vi "Nufern Functional Global.vi"(4 "Galvo.lvclass":refnum<class "Galvo.lvclass">, 7 "Nufern Functional\n Global States":T2, 8 "Error In":errorcluster, 10 "Nufern Digital Timing Control":T1={"Fire"=FALSE, "Start A-Scan"=0, "Stop A-Scan"=0, "Reps per Fire"=1, "B-Scan Spacing"=1} {"B-Scan Spacing" min=0 max=5000; "Reps per Fire" min=1 max=5000}) -> (0 "Error Out":errorcluster)   [LabVIEW 2015]
uses:
  Nufern Functional Global States.ctl
  Galvo/Galvo.lvclass
  Nufern Digital Timing Control.ctl
  NuFern.lvclass
  DIO/NIDIO/NIDIO.lvclass
panel:
  out "Waveform Graph":dbl[][](graph)
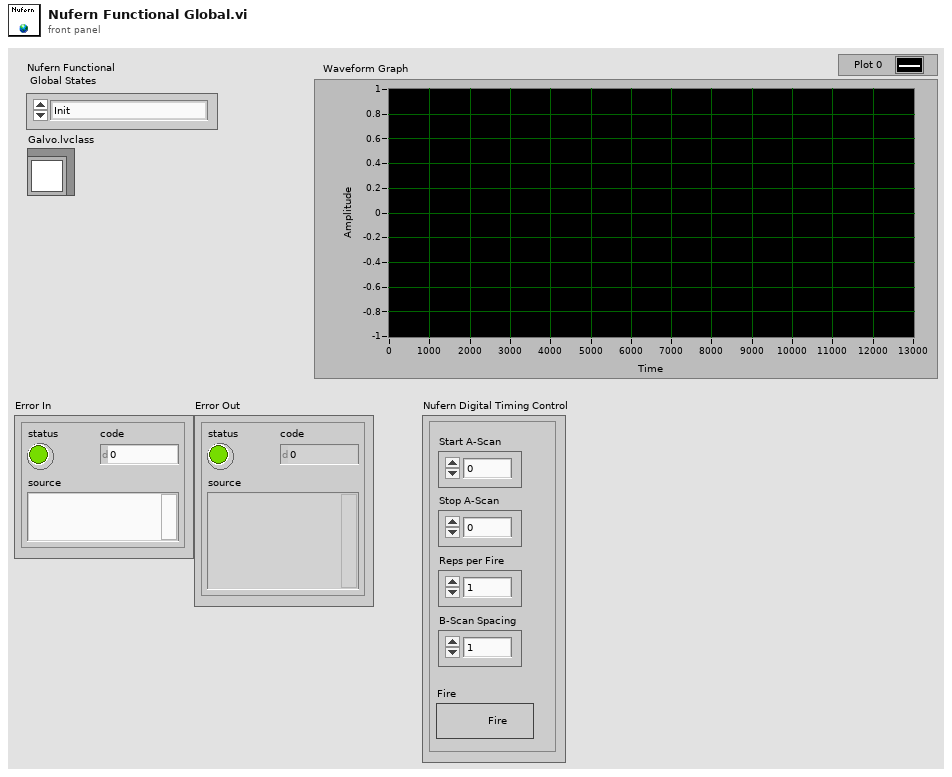
[diagram p1: front panel]
types:
  T1 = typedef "Nufern Digital Timing Control.ctl" = cluster{"Fire":bool, "Start A-Scan":u32, "Stop A-Scan":u32, "Reps per Fire":i32, "B-Scan Spacing":i32}
  T2 = typedef "Nufern Functional Global States.ctl" = enum16{"Init", "Generate Waveform", "Fire", "Shutdown", "Stop"}
  T3 = typedef "DAQ Class.lvclass/DAQ Parameters.ctl" = cluster{"Points Per A-Scan":u32, "A-Scans Per B-Scan":u32, "Number of B-Scans":u32, "B-Scans Per Transfer":u32, "Trigger Voltage":sgl, "Trigger Source":T4, "Trigger Slope":T5, "Channel":T6, "Clock":T7, "Bits per Sample":dbl, "Range":dbl, "Start Trim":u32, "Stop Trim":u32}
  T4 = typedef "DAQ Class.lvclass/Trigger Source.ctl" = enum16{"External", "Channel A", "Channel B"}
  T5 = typedef "DAQ Class.lvclass/Trigger Slope.ctl" = enum16{"Rising", "Falling"}
  T6 = typedef "OCT DAQ Channel Data Type.ctl" = enum16{"Channel 1", "Channel 2", "Channel 1 and 2"}
  T7 = typedef "DAQ Class.lvclass/Clock Control.ctl" = enum16{"Internal Clock", "External Clock"}
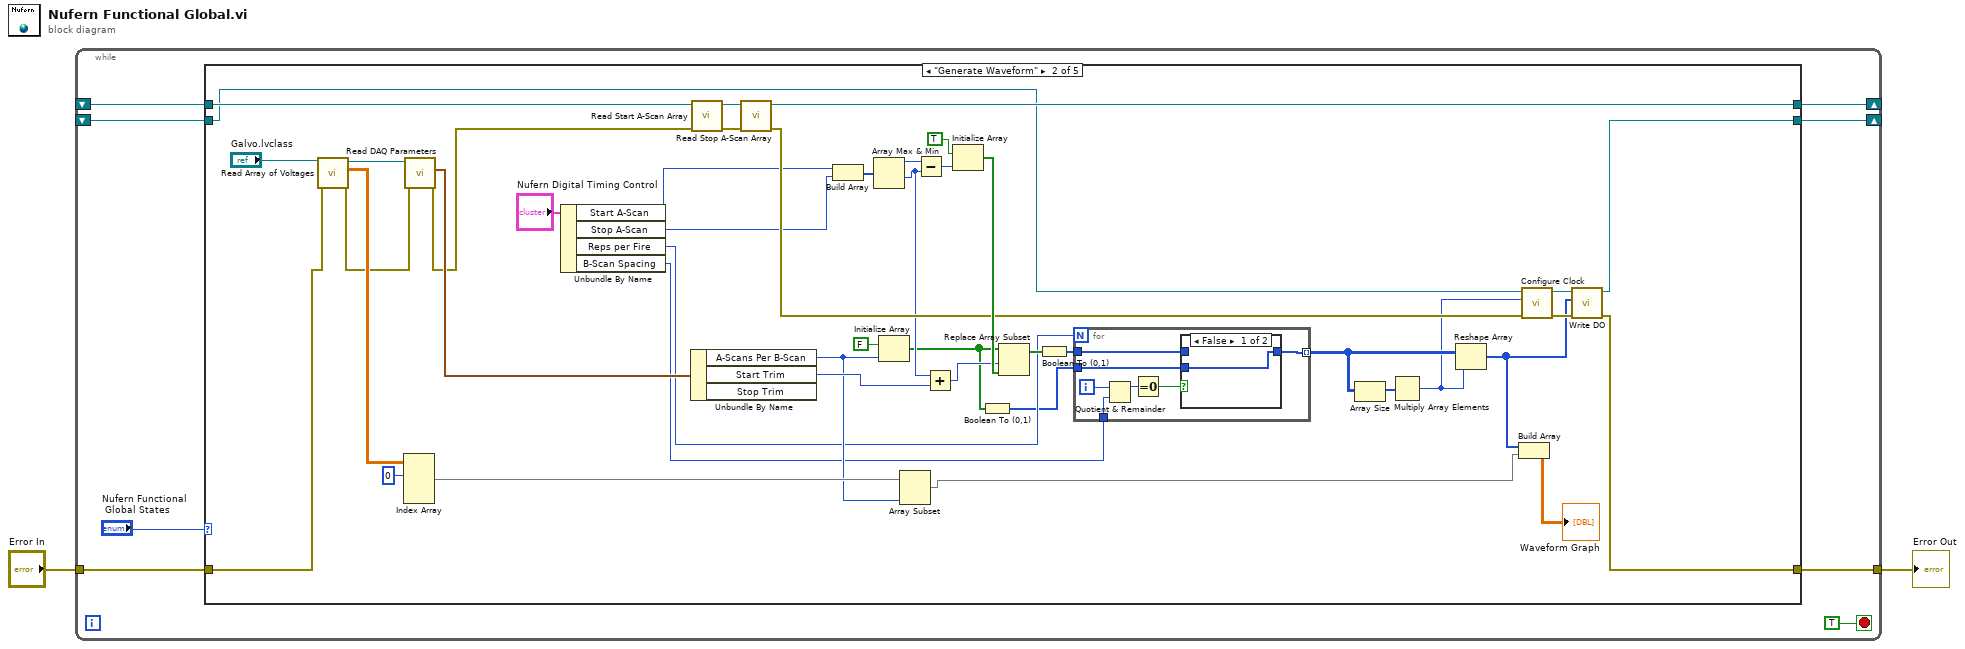
[diagram p0: block diagram]
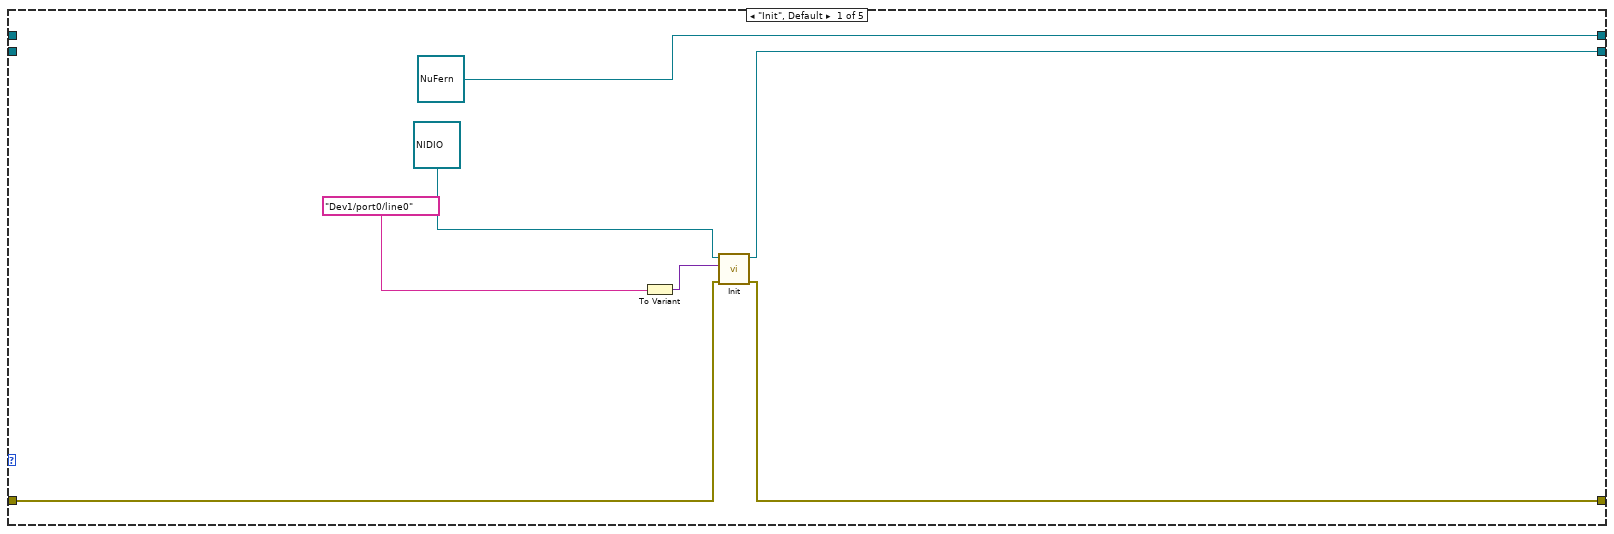
[diagram p2: hidden frame]
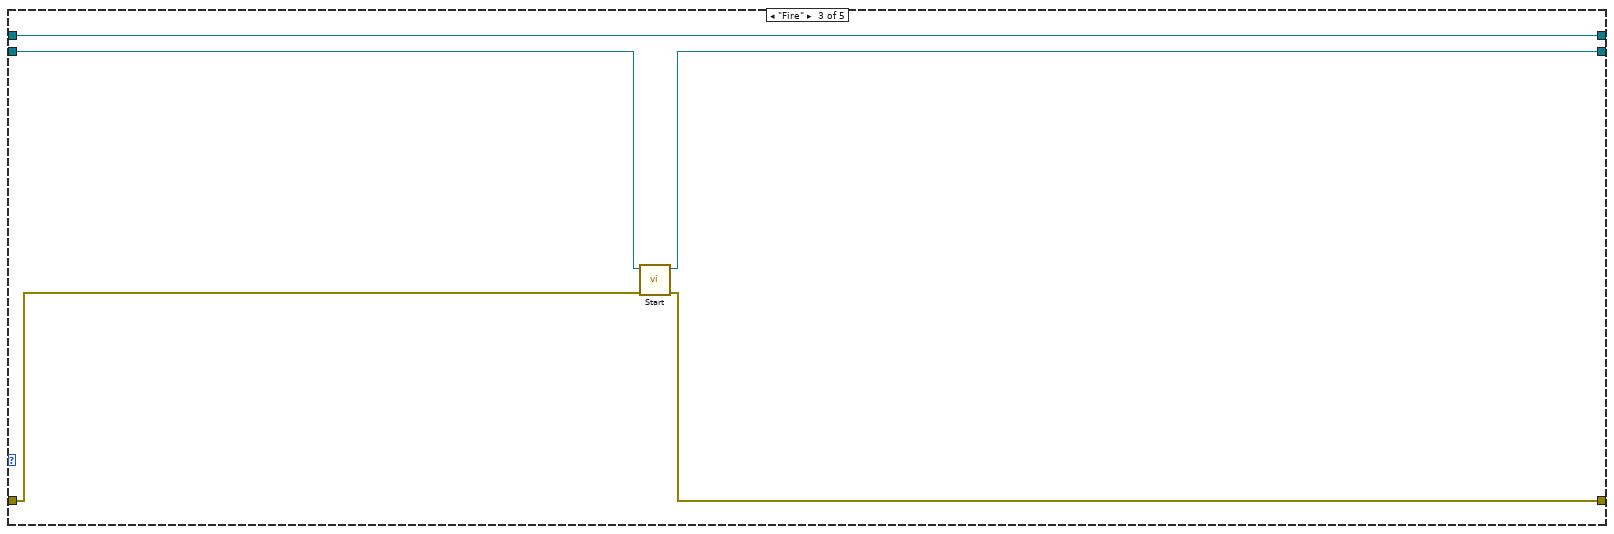
[diagram p4: hidden frame]
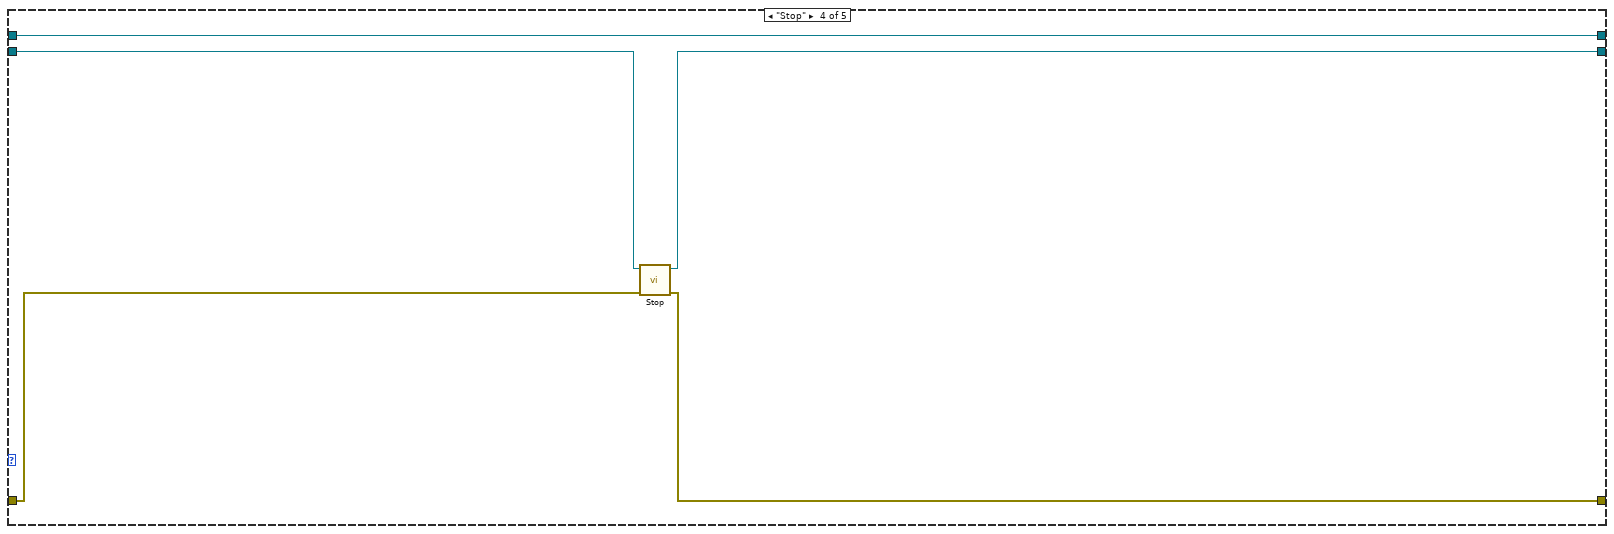
[diagram p5: hidden frame]
diagram:
  n1 = while {
    shift-right: [w7] -> _
    shift-left: _ -> [w9]
    tunnel: "Error In" -> [w6]
    tunnel: [w5] -> w1
    shift-right: [w3] -> _
    shift-left: _ -> [w4]
    stop <- TRUE stop-if-true
    n2 = case shown="\"Generate Waveform\"" "Nufern Functional\n Global States" {
      tunnel: w9 -> [_ w54 w75 w80 w83]
      tunnel: [refnum<class "NuFern.lvclass"> refnum ("NuFern.lvclass") w51 w75 w80 w83] -> w7
      tunnel: w6 -> [w11 w60 w72 w77 w82]
      tunnel: [w13 w38 w71 w76 w82] -> w5
      tunnel: w4 -> [_ w43 w74 w79 w81]
      tunnel: [w15 w39 w73 w78 w81] -> w3
      frame "Init", Default {
        n3 = To Variant(anything=tag "Dev1/port0/line0" ("lines")) -> (Variant=w14:variant)
        n4 = call-dynamic "Init.vi"("error in (no error)"=w11, "DIO Configuration In"=w14, "NIDIO in"=refnum<class "NIDIO.lvclass"> refnum ("NIDIO.lvclass")) -> ("error out"=w13:errorcluster, "NIDIO out"=w15:refnum<class "NIDIO.lvclass">)  [unwired: 7 in]
      }
      frame "Generate Waveform" {
        n5 = call-dynamic "Read Array of Voltages.vi"("error in (no error)"=w60, "Galvo in"="Galvo.lvclass") -> ("error out"=w56:errorcluster, "Array of Voltages"=w59:dbl[][], "Galvo out"=w57:refnum<class "Galvo.lvclass">)  [unwired: 7 in]
        n6 = Index Array(array=w59, index (row) #1=0 ("index (row)")) -> (element #1=w33:dbl[])  [unwired: 3 in, 1 out]
        n7 = call-dynamic "Read DAQ Parameters.vi"("error in (no error)"=w56, "Galvo in"=w57) -> ("error out"=w50:errorcluster, "DAQ Parameters"=w55:T3)  [unwired: 7 in, 1 out]
        n8 = Unbundle By Name("Nufern Digital Timing Control") -> ("Start A-Scan"=w28:u32, "Stop A-Scan"=w27:u32, "Reps per Fire"=w25:i32, "B-Scan Spacing"=w20:i32)
        n9 = Unbundle By Name(w55) -> ("A-Scans Per B-Scan"=w31:u32, "Start Trim"=w34:u32)  [unwired: 1 out]
        n10 = call-dynamic "Read Start A-Scan Array.vi"("error in (no error)"=w50, "NuFern in"=w54) -> ("error out"=w52:errorcluster, "NuFern out"=w53:refnum<class "NuFern.lvclass">)  [unwired: 7 in, 1 out]
        n11 = call-dynamic "Read Stop A-Scan Array.vi"("error in (no error)"=w52, "NuFern in"=w53) -> ("error out"=w42:errorcluster, "NuFern out"=w51:refnum<class "NuFern.lvclass">)  [unwired: 7 in, 1 out]
        n12 = Build Array(w28, w27) -> (w48:u32[])
        n13 = Array Max & Min(array=w48) -> (max value=w47:u32, min value=w35:u32)  [unwired: 2 out]
        n14 = Initialize Array(FALSE, w31) -> (w19:bool[])
        n15 = Array Subset(array=w33, length=w31) -> (w32:dbl[])  [unwired: 1 in]
        n16 = Subtract(x=w47, y=w35) -> (x-y=w46:u32)
        n17 = Add(x=w35, y=w34) -> (x+y=w36:u32)
        n18 = Initialize Array(TRUE, w46) -> (w44:bool[])
        n19 = Boolean To (0,1)(Boolean=w19) -> (0, 1=w18:i16[])
        n20 = Replace Array Subset(array=w19, new element=w44, index=w36) -> (w40:bool[])
        n21 = Boolean To (0,1)(Boolean=w40) -> (0, 1=w26:i16[])
        n22 = for {
          N: w25 -> [_]
          tunnel: w26 -> [w63]
          tunnel: [w64] -> w24 mode=indexing
          tunnel: w20 -> [w67]
          tunnel: w18 -> [w62]
          i -> [w68]
          n23 = Quotient & Remainder(x=w68, y=w67) -> (x-y*floor(x/y)=w66:i32)  [unwired: 1 out]
          n24 = Equal To 0?(x=w66) -> (x = 0?=w65:bool)
          n25 = case shown="False" w65 {
            tunnel: [w69 w70] -> w64
            tunnel: w63 -> [_ w70]
            tunnel: w62 -> [w69 _]
            frame False {
            }
            frame True {
            }
          }
        }
        n26 = Array Size(array=w24) -> (size(s)=w23:i32[])
        n27 = Multiply Array Elements(1:w23) -> (0:w21:i32)
        n28 = Reshape Array(w24, w21) -> (w22:i16[])
        n29 = Build Array(w22, w32) -> (→"Waveform Graph":dbl[][])
        n30 = call-dynamic "Configure Clock.vi"("error in (no error)"=w42, "samples per channel"=w21, "NIDIO in"=w43) -> ("error out"=w37:errorcluster, "NIDIO out"=w41:refnum<class "NIDIO.lvclass">)  [unwired: 7 in]
        n31 = call-dynamic "Write DO.vi"("error in (no error)"=w37, "Array"=w22, "NIDIO in"=w41) -> ("error out"=w38:errorcluster, "NIDIO out"=w39:refnum<class "NIDIO.lvclass">)  [unwired: 7 in]
      }
      frame "Fire" {
        n32 = call-dynamic "Start.vi"("error in (no error)"=w72, "NIDIO in"=w74) -> ("error out"=w71:errorcluster, "NIDIO out"=w73:refnum<class "NIDIO.lvclass">)  [unwired: 8 in]
      }
      frame "Stop" {
        n33 = call-dynamic "Stop.vi"("error in (no error)"=w77, "NIDIO in"=w79) -> ("error out"=w76:errorcluster, "NIDIO out"=w78:refnum<class "NIDIO.lvclass">)  [unwired: 8 in]
      }
      frame "Shutdown" {
      }
    }
  }
  "Error Out" <- w1
